vi "Open Wrapper.vi"(8 "error in (no error)":errorcluster, 11 "Configuration Json":string) -> (0 "error out":errorcluster, 3 "Session":u64)   [LabVIEW 2021, in "Zenoh.lvclass"]
uses:
  Zenoh.lvclass
  typedef/Zenoh Errors.ctl
  <vilib>/CIF Foundation/CIF Utilities/Errors/Append Error Location.vi
  Zenoh.lvclass/Zenoh.ctl
  <vilib>/CIF Foundation/CIF Utilities/File/File_CIF_U.lvlib
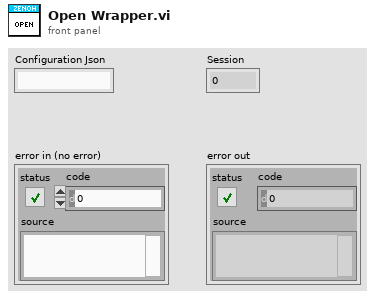
[diagram p1: front panel]
types:
  T1 = typedef "Zenoh.lvclass/Zenoh Errors.ctl" = enum16{"Open Session Error", "Open Subscription Error", "Declare Liveliness", "Query Keys", "File Error", "JSON Error", "Zenoh Runtime"}
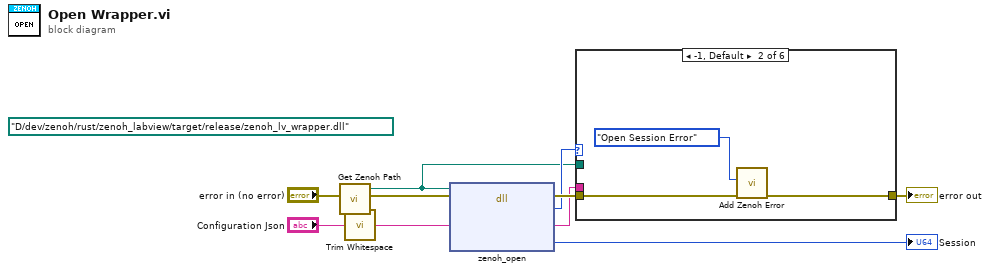
[diagram p0: block diagram]
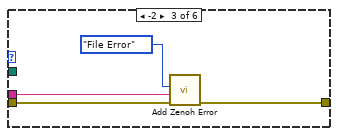
[diagram p3: hidden frame]
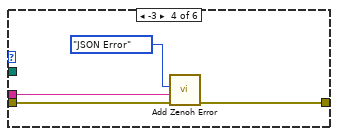
[diagram p4: hidden frame]
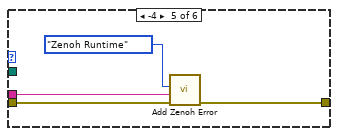
[diagram p5: hidden frame]
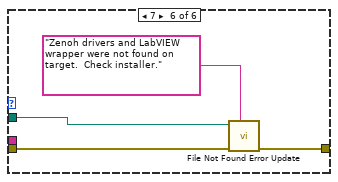
[diagram p6: hidden frame]
diagram:
  (unwired) path "D:/dev/zenoh/rust/zenoh_labview/target/release/zenoh_lv_wrapper.dll" ("path in")
  n1 = call "Get Zenoh Path.vi"() -> ("Library Path"=w1:path)  [unwired: 4 in]
  n2 = call <vilib>:"Trim Whitespace.vi"("string"="Configuration Json") -> ("trimmed string"=w2:string)  [unwired: 1 in]
  n3 = dll-call lib="C:/Program Files/CIF_Foundation/Libraries/zenoh_lv_wrapper.dll" fn="zenoh_open"(path in=w1, error in="error in (no error)", "config_input"=w2) -> (error out=w8:errorcluster, "Return Value"=w4:i32, "config_input"=w3:string, "session_out"=→"Session":u64)  [unwired: 2 in, 1 out]
  n4 = case shown="-1, Default" w4 {
    tunnel: w8 -> [w10 w13 w17 w21 w25 w29]
    tunnel: [w10 w12 w16 w20 w24 w28] -> w7
    tunnel: w3 -> [_ _ w14 w18 w22 _]
    tunnel: w1 -> [_ _ _ _ _ w27]
    frame 0 {
    }
    frame -1, Default {
      n5 = call "Add Zenoh Error.vi"("error in (no error)"=w13, "Error"=Zenoh_Errors."Open Session Error") -> ("error out"=w12:errorcluster)  [unwired: 9 in]
    }
    frame -2 {
      n6 = call "Add Zenoh Error.vi"("error in (no error)"=w17, "String to Append"=w14, "Error"=Zenoh_Errors."File Error") -> ("error out"=w16:errorcluster)  [unwired: 8 in]
    }
    frame -3 {
      n7 = call "Add Zenoh Error.vi"("error in (no error)"=w21, "String to Append"=w18, "Error"=Zenoh_Errors."JSON Error") -> ("error out"=w20:errorcluster)  [unwired: 8 in]
    }
    frame -4 {
      n8 = call "Add Zenoh Error.vi"("error in (no error)"=w25, "String to Append"=w22, "Error"=Zenoh_Errors."Zenoh Runtime") -> ("error out"=w24:errorcluster)  [unwired: 8 in]
    }
    frame 7 {
      n9 = call <vilib>:"File Not Found Error Update.vi"("Custom Message"="Zenoh drivers and LabVIEW wrapper were not found on target.  Check installer.", "error in"=w29, "path in"=w27) -> ("error out"=w28:errorcluster)  [unwired: 8 in]
    }
  }
  "error out" <- w7
